vi "GetSlopeConductance2.vi"(9 "CapacitanceRecords":T2[](array[typedef]), 11 "Array in":dbl[][](array[numeric])) -> (2 "parameters":T1, 3 "FitView":cluster{dbl[], dbl[]}[](array[cluster]))   [LabVIEW 2020]
uses:
  CapacitanceRecord.ctl
  <vilib>/Analysis/6fits.llb/Curve Fitting Criteria.ctl
  <vilib>/Analysis/NI_AALPro.lvlib
panel:
  out "XY Graph":cluster{dbl[], dbl[]}[](graph)
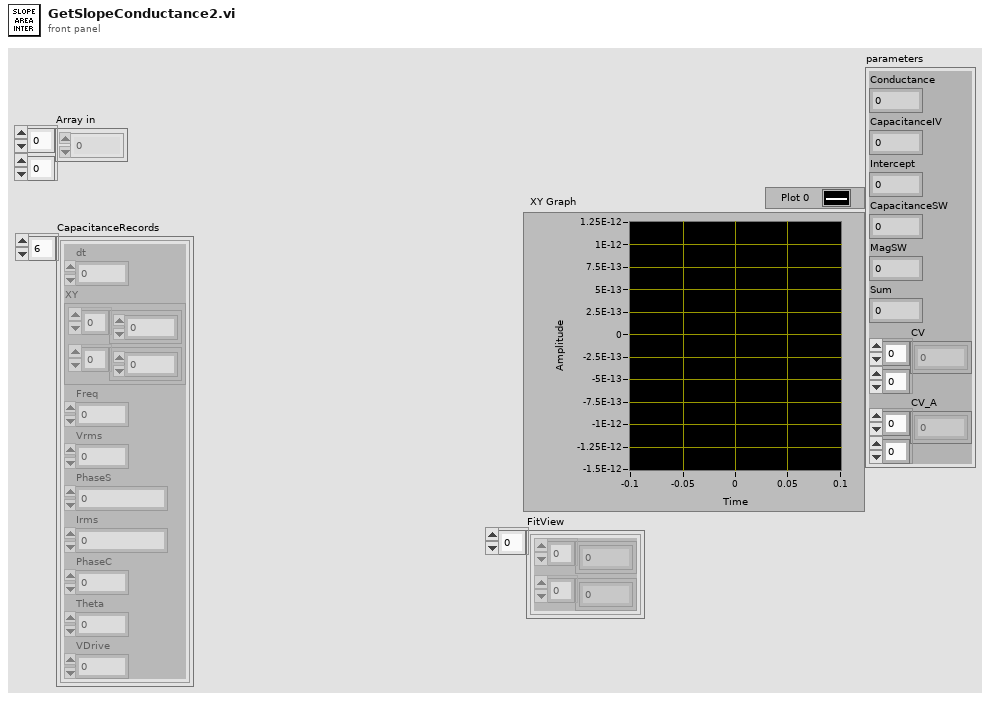
[diagram p1: front panel]
types:
  T1 = cluster{"Conductance":dbl, "CapacitanceIV":dbl, "Intercept":dbl, "CapacitanceSW":dbl, "MagSW":dbl, "Sum":dbl, "CV":dbl[][], "CV_A":dbl[][]}
  T2 = typedef "CapacitanceRecord.ctl" = cluster{"dt":dbl, "XY":cluster{dbl[], dbl[]}, "Freq":dbl, "Vrms":dbl, "PhaseS":dbl, "Irms":dbl, "PhaseC":dbl, "Theta":dbl, "VDrive":dbl}
  T3 = typedef "NI_AALPro.lvlib/Curve Fitting Criteria.ctl" = u16
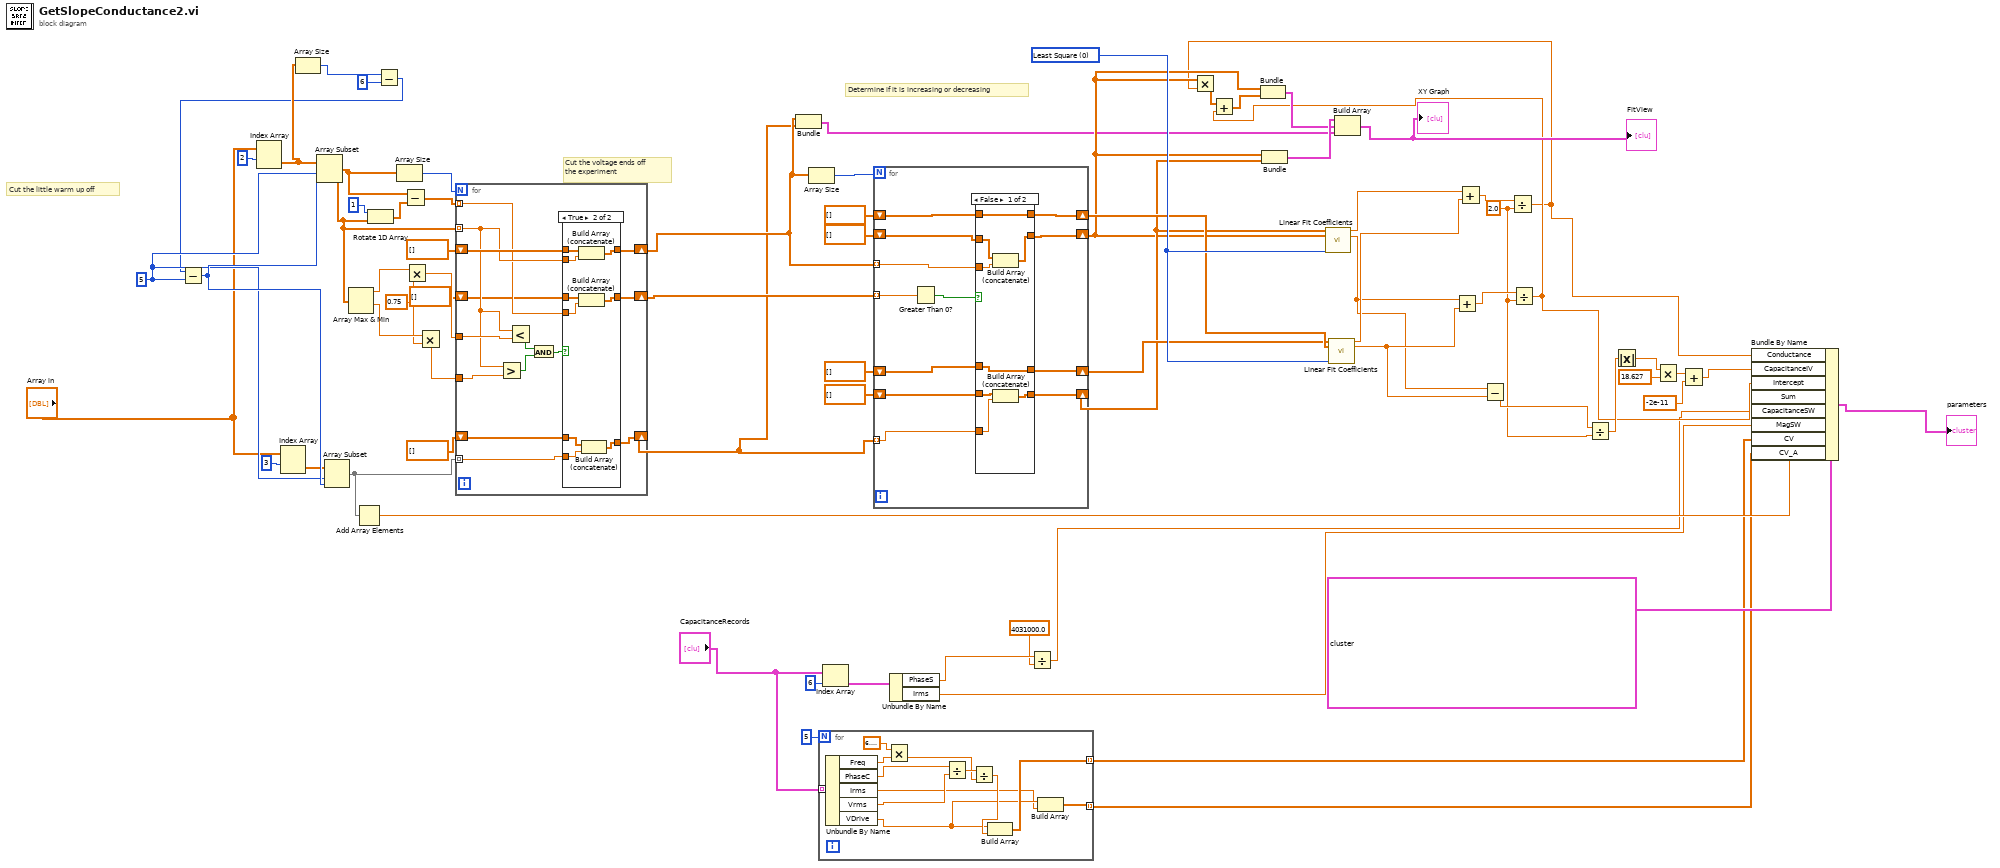
[diagram p0: block diagram]
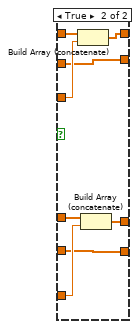
[diagram p2: hidden frame]
diagram:
  w46 = 2.0 ("y")
  w65 = 0.75 ("y")
  w71 = 5 ("y")
  w60 = T3 0 items=["Least Square", "Least Absolute Residual", "Bisquare"] ("method")
  # "Determine if it is increasing or decreasing"
  # "Cut the little warm up off"
  # "Cut the voltage ends off\nthe experiment"
  n1 = Index Array(array="Array in", index (row)=2) -> (element=w44:dbl[])  [unwired: 1 in]
  n2 = Index Array(array="Array in", index (row)=3) -> (element=w68:dbl[])  [unwired: 1 in]
  n3 = Array Size(array=w44) -> (size(s)=w43:i32)
  n4 = Subtract(x=w43, y=6) -> (x-y=w41:i32)
  n5 = Subtract(x=w41, y=w71) -> (x-y=w72:i32)
  n6 = Array Subset(array=w44, index=w71, length=w72) -> (w56:dbl[])
  n7 = Array Subset(array=w68, index=w71, length=w72) -> (w59:dbl[])
  n8 = Array Max & Min(array=w56) -> (max value=w67:dbl, min value=w66:dbl)  [unwired: 2 out]
  n9 = Add Array Elements(numeric array=w59) -> (sum=w16:dbl)
  n10 = Rotate 1D Array(1:w56, 2:1 ("n")) -> (0:w57:dbl[])
  n11 = Array Size(array=w56) -> (size(s)=w64:i32)
  n12 = Subtract(x=w56, y=w57) -> (x-y=w55:dbl[])
  n13 = Multiply(x=w67, y=w65) -> (x*y=w63:dbl)
  n14 = Multiply(x=w66, y=w65) -> (x*y=w62:dbl)
  n15 = for {
    N: w64 -> [_]
    tunnel: w56 -> [w79] mode=indexing
    tunnel: w59 -> [w78] mode=indexing
    tunnel: w63 -> [w83]
    tunnel: w62 -> [w82]
    shift-right: [w80] -> w23
    shift-left: dbl[] [] -> [w81]
    shift-right: [w77] -> w22
    shift-left: dbl[] [] -> [w76]
    tunnel: w55 -> [w75] mode=indexing
    shift-right: [w74] -> w54
    shift-left: dbl[] [] -> [w73]
    n16 = Greater?(x=w79, y=w82) -> (0:w84:bool)
    n17 = Less?(x=w79, y=w83) -> (x < y?=w86:bool)
    n18 = And(x=w86, y=w84) -> (x .and. y?=w85:bool)
    n19 = case shown="True" w85 {
      tunnel: w81 -> [w89 w97]
      tunnel: [w89 w98] -> w80
      tunnel: w79 -> [_ w96]
      tunnel: w78 -> [_ w95]
      tunnel: [w88 w94] -> w77
      tunnel: w76 -> [w88 w93]
      tunnel: w75 -> [_ w92]
      tunnel: [w87 w91] -> w74
      tunnel: w73 -> [w87 w90]
      frame False {
      }
      frame True {
        n20 = Build Array (concatenate)(w97, w96) -> (w98:dbl[])
        n21 = Build Array (concatenate)(w90, w92) -> (w91:dbl[])
        n22 = Build Array (concatenate)(w93, w95) -> (w94:dbl[])
      }
    }
  }
  n23 = Bundle(w23, w22) -> (w21:cluster{dbl[], dbl[]})  [unwired: 1 in]
  n24 = Array Size(array=w23) -> (size(s)=w61:i32)
  n25 = for {
    N: 5 -> [_]
    tunnel: "CapacitanceRecords" -> [w110] mode=indexing
    tunnel: [w99] -> w2 mode=indexing
    tunnel: [w102] -> w3 mode=indexing
    n26 = Unbundle By Name(w110) -> ("Freq"=w106:dbl, "PhaseC"=w109:dbl, "Irms"=w100:dbl, "Vrms"=w108:dbl, "VDrive"=w101:dbl)
    n27 = Multiply(x=6.283185307179586, y=w106) -> (x*y=w105:dbl)
    n28 = Divide(x=w109, y=w108) -> (x/y=w107:dbl)
    n29 = Divide(x=w107, y=w105) -> (x/y=w103:dbl)
    n30 = Build Array(w101, w103) -> (w102:dbl[])
    n31 = Build Array(w101, w100) -> (w99:dbl[])
  }
  n32 = Index Array(array="CapacitanceRecords", index=6) -> (element=w10:T2)
  n33 = for {
    N: w61 -> [_]
    tunnel: w23 -> [w120] mode=indexing
    tunnel: w54 -> [w119] mode=indexing
    shift-right: [w121] -> w53
    shift-left: dbl[] [] -> [w122]
    shift-right: [w111] -> w26
    shift-left: dbl[] [] -> [w112]
    shift-right: [w113] -> w52
    shift-left: dbl[] [] -> [w114]
    shift-right: [w117] -> w29
    shift-left: dbl[] [] -> [w116]
    tunnel: w22 -> [w115] mode=indexing
    n34 = Greater Than 0?(x=w119) -> (x > 0?=w118:bool)
    n35 = case shown="False" w118 {
      tunnel: w122 -> [w130 w137]
      tunnel: [w130 w138] -> w121
      tunnel: w120 -> [w125 w136]
      tunnel: w115 -> [w124 w135]
      tunnel: [w129 w131] -> w111
      tunnel: [w128 w134] -> w117
      tunnel: w116 -> [w126 w134]
      tunnel: w112 -> [w127 w131]
      tunnel: w114 -> [w123 w133]
      tunnel: [w123 w132] -> w113
      frame False {
        n36 = Build Array (concatenate)(w127, w125) -> (w129:dbl[])
        n37 = Build Array (concatenate)(w126, w124) -> (w128:dbl[])
      }
      frame True {
        n38 = Build Array (concatenate)(w137, w136) -> (w138:dbl[])
        n39 = Build Array (concatenate)(w133, w135) -> (w132:dbl[])
      }
    }
  }
  n40 = Unbundle By Name(w10) -> ("PhaseS"=w8:dbl, "Irms"=w9:dbl)
  n41 = Divide(x=w8, y=4031000.0) -> (x/y=w6:dbl)
  n42 = Bundle(w26, w29) -> (w32:cluster{dbl[], dbl[]})  [unwired: 1 in]
  n43 = call <vilib>:"Linear Fit Coefficients.vi"("Y"=w29, "X"=w26, "method"=w60) -> ("slope"=w25:dbl, "intercept"=w24:dbl)  [unwired: 10 in, 1 out]
  n44 = call <vilib>:"Linear Fit Coefficients.vi"("Y"=w52, "X"=w53, "method"=w60) -> ("slope"=w51:dbl, "intercept"=w48:dbl)  [unwired: 10 in, 1 out]
  n45 = Add(x=w24, y=w48) -> (x+y=w49:dbl)
  n46 = Add(x=w25, y=w51) -> (x+y=w50:dbl)
  n47 = Subtract(x=w24, y=w48) -> (x-y=w47:dbl)
  n48 = Divide(x=w50, y=w46) -> (x/y=w17:dbl)
  n49 = Multiply(x=w26, y=w17) -> (x*y=w28:dbl[])
  n50 = Divide(x=w49, y=w46) -> (x/y=w18:dbl)
  n51 = Add(x=w28, y=w18) -> (x+y=w27:dbl[])
  n52 = Bundle(w26, w27) -> (w31:cluster{dbl[], dbl[]})  [unwired: 1 in]
  n53 = Build Array(w32, w31, w21) -> (→"XY Graph" →"FitView":cluster{dbl[], dbl[]}[])
  n54 = Divide(x=w47, y=w46) -> (x/y=w45:dbl)
  n55 = Absolute Value(x=w45) -> (abs(x)=w20:dbl)
  n56 = Multiply(x=w20, y=18.627) -> (x*y=w15:dbl)
  n57 = Add(x=w15, y=-2e-11) -> (x+y=w13:dbl)
  n58 = Bundle By Name(cluster=T1 {"Conductance"=0.0, "CapacitanceIV"=0.0, "Intercept"=0.0, "CapacitanceSW"=0.0, "MagSW"=0.0, "Sum"=0.0, "CV"=array4x400[1600 elements], "CV_A"=array4x400[1600 elements]}, "Conductance"=w17, "CapacitanceIV"=w13, "Intercept"=w18, "Sum"=w16, "CapacitanceSW"=w6, "MagSW"=w9, "CV"=w3, "CV_A"=w2) -> (→"parameters":T1)
